vi "TCP Write.vi"(8 "error in (no error)":errorcluster, 9 "timeout ms (25000)":i32=25000, 10 "data in":string, 11 "TCP in":refnum<class "TCP.lvclass">) -> (0 "error out":errorcluster, 2 "bytes written":i32, 3 "TCP out":refnum<class "TCP.lvclass">)   [LabVIEW 2013, in "TCP.lvclass"]
doc: "Writes data to a TCP network connection"
uses:
  TCP.lvclass
  TCP.lvclass/TCP.ctl
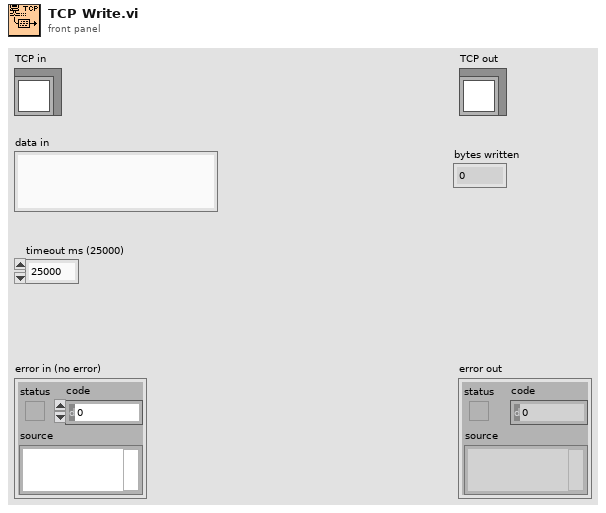
[diagram p1: front panel]
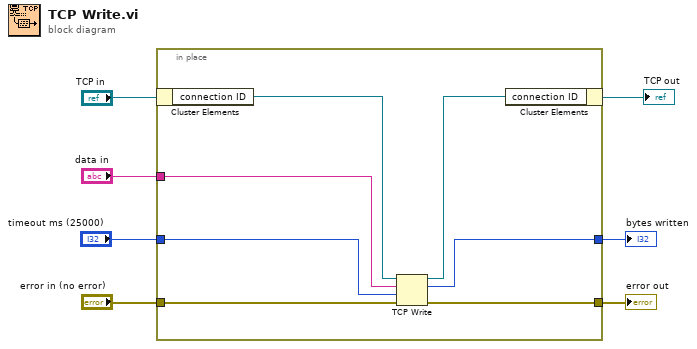
[diagram p0: block diagram]
diagram:
  n1 = in-place {
    in-place-border: "error in (no error)" -> [w12]
    in-place-border: "data in" -> [w11]
    in-place-border: "timeout ms (25000)" -> [w10]
    in-place-border: [w9] -> w2
    in-place-border: [w8] -> w1
    n2 = in-place-cluster #1("TCP in") -> ("connection ID"=w14:refnum<k5>)
    n3 = TCP Write(connection ID=w14, data in=w11, error in (no error)=w12, 9:w10) -> (connection ID out=w13:refnum<k5>, bytes written=w9:i32, error out=w8:errorcluster)
    n4 = in-place-cluster #1("connection ID"=w13) -> (→"TCP out":refnum<class "TCP.lvclass">)
  }
  "error out" <- w1
  "bytes written" <- w2
